vi "startup.vi"(8 "error in (no error)":errorcluster, 11 "Boot in":refnum<class "Boot.lvclass">) -> (0 "error out":errorcluster, 3 "Boot out":refnum<class "Boot.lvclass">)   [LabVIEW 2016, in "Boot.lvclass"]
uses:
  Boot.lvclass
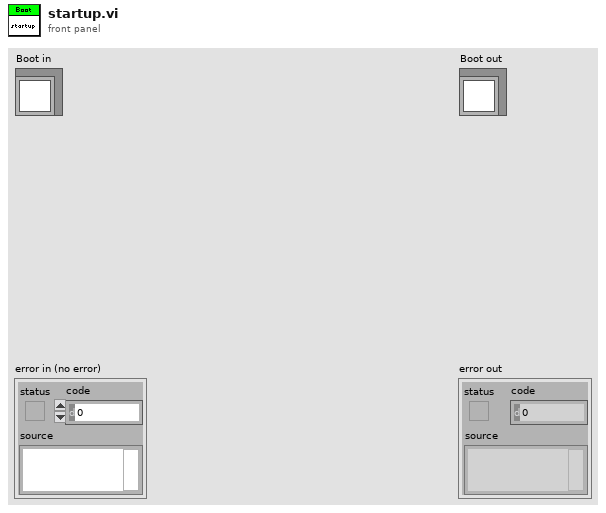
[diagram p1: front panel]
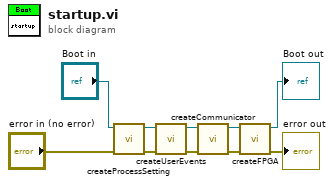
[diagram p0: block diagram]
diagram:
  n1 = call "createProcessSetting.vi"("error in (no error)"="error in (no error)", "Boot in"="Boot in") -> ("error out"=w5:errorcluster, "Boot out"=w9:refnum<class "Boot.lvclass">)  [unwired: 7 in, 1 out]
  n2 = call "createUserEvents.vi"("error in (no error)"=w5, "Boot in"=w9) -> ("error out"=w4:errorcluster, "Boot out"=w8:refnum<class "Boot.lvclass">)  [unwired: 7 in, 1 out]
  n3 = call "createCommunicator.vi"("error in (no error)"=w4, "Boot in"=w8) -> ("error out"=w3:errorcluster, "Boot out"=w7:refnum<class "Boot.lvclass">)  [unwired: 7 in, 1 out]
  n4 = call "createFPGA.vi"("error in (no error)"=w3, "Boot in"=w7) -> ("error out"=→"error out":errorcluster, "Boot out"=→"Boot out":refnum<class "Boot.lvclass">)  [unwired: 7 in, 1 out]
